vi "Robot Global Data.vi"() -> ()   [LabVIEW 2017]
doc: "This global VI can contain as many global variables as you need. Place a control on the panel, give it a good name. To read or write to it from a VI, drag the icon to the diagram of that VI. You can also drag from the project. Click on the node to change which global you access. You shouldn't have multiple locations writing to a global or it will cause a race-condition."
uses:
  <vilib>/Rock Robotics/WPI/Camera/WPI_CameraImageSize.ctl
  <vilib>/Rock Robotics/WPI/DriverStation/WPI_DriverStationRobotMode2.ctl
  Auto.ctl
  RobotPosition.ctl
  typedef/Encoder.ctl
  DriveMode.ctl
panel:
  in  "GyroRange":dbl
  in  "DriveMode":T1
  in  "Encoder":T2
  in  "RobotPosition":T3
  in  "FAutoGyro":dbl
  in  "DAutoGyro":dbl
  in  "IAutoGyro":dbl
  in  "PAutoGyro":dbl=0.0003
  in  "MoProAlmostDone":bool
  in  "MoProDone":bool
  in  "XYRatio":dbl
  in  "PigeonTimeout":dbl
  in  "PigeonAngleDif":dbl
  in  "DriveStraight":bool
  in  "MaxRPM":dbl=1000.0
  in  "RampRateAuto":dbl=1.0
  in  "RampRateTele":dbl=1.0
  in  "AutoDelay":dbl
  in  "Logging":bool
  in  "Inverse":bool
  in  "FTeleGyro":dbl
  in  "DTeleGyro":dbl
  in  "ITeleGyro":dbl
  in  "PTeleGyro":dbl=0.0003
  in  "FTeleLeft":dbl
  in  "FTeleRight":dbl
  in  "DAuto":dbl
  in  "FAutoLeft":dbl
  in  "FAutoRight":dbl
  in  "PAuto":dbl
  in  "IAuto":dbl
  in  "DTele":dbl
  in  "ITele":dbl
  in  "PTele":dbl
  in  "TurboPercent":dbl=1.0
  in  "NormalPercent":dbl=0.5
  in  "Autonomous":T4
  in  "Gyro":bool
  in  "Robot Mode":T5
  in  "image size":T6=enum."320x240"
  in  "Enable Vision":bool
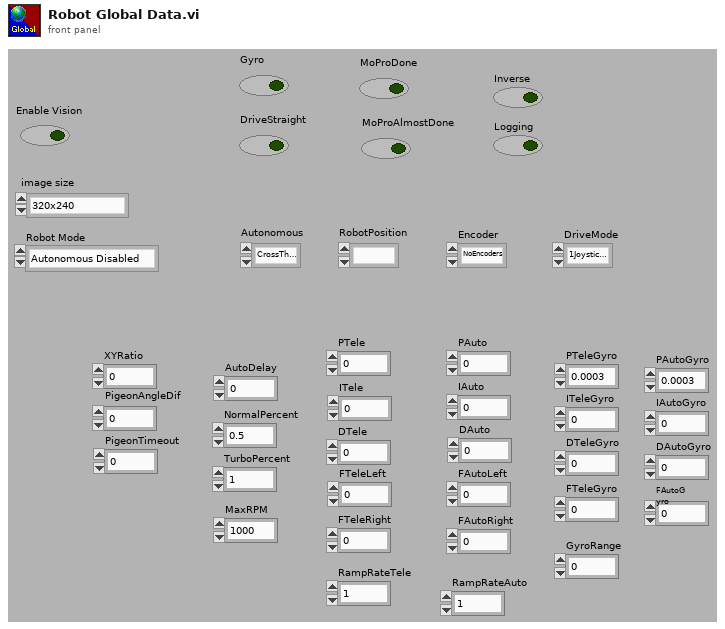
[diagram p1: front panel]
types:
  T1 = typedef "DriveMode.ctl" = enum16{"1JoystickArcade", "2JoystickArcade", "Tank"}
  T2 = typedef "Encoder.ctl" = enum16{"NoEncoders", "ShaftEncoders", "MotorEncoders"}
  T3 = typedef "RobotPosition.ctl" = enum16{""}
  T4 = typedef "Auto.ctl" = enum16{"CrossTheLine", "DoNothing"}
  T5 = typedef "WPI_DriverStationRobotMode2.ctl" = enum16{"Autonomous Disabled", "Autonomous Enabled", "Teleop Disabled", "Teleop Enabled", "Disconnected", "Finish", "Test Disabled", "Test Enabled", "Emergency Stopped"}
  T6 = typedef "WPI_CameraImageSize.ctl" = enum16{"640x480", "320x240", "160x120", "Custom"}
diagram:
